vi "AnalysisProcess.vi"(7 "RestartBlocksStates?":bool, 8 "error in (no error)":errorcluster, 9 "Tacho signal In":waveform(dbl), 10 "AccelerationDataIn":waveform(dbl)[](array[waveform]), 11 "QueuesIn":T1) -> (0 "error out":errorcluster, 2 "Tacho signal Out out":waveform(dbl), 3 "AccelerationDataOut out":waveform(dbl)[](array[waveform]))   [LabVIEW 2019]
uses:
  utilities/AQueues.ctl
  AmasterVIs/ACommand.ctl
  AnalyzedVibrationsData.ctl
  AccelerationDataFrames.ctl
  calculateFaultIndicatorsVIs/FaultDetections.ctl
  calculateFaultIndicatorsVIs/ParameterFaultDetection.ctl
  calculateFaultIndicatorsVIs/FaultParameter.ctl
  calculateFaultIndicatorsVIs/FrequencyFaultDetection.ctl
  calculateFaultIndicatorsVIs/OrdersFaultDetection.ctl
  TDMSmanagerVIs/TDMSAnalyzerData.ctl
  TDMSmanagerVIs/TDMSAnalyzerDataType.ctl
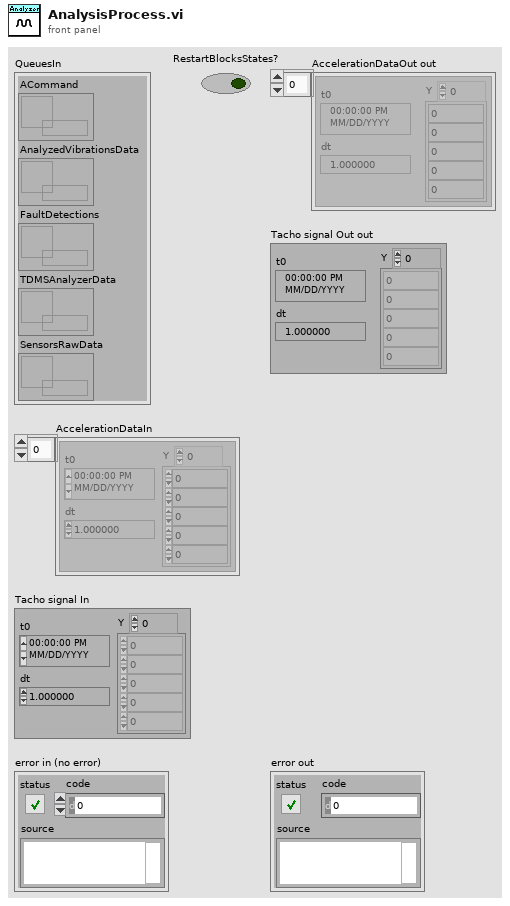
[diagram p1: front panel]
types:
  T1 = typedef "AQueues.ctl" = cluster{"ACommand":refnum<queue>, "AnalyzedVibrationsData":refnum<queue>, "FaultDetections":refnum<queue>, "TDMSAnalyzerData":refnum<queue>, "SensorsRawData":refnum<queue>}
  T2 = typedef "AnalyzerSettings.ctl" = cluster{"Create NS Timeout Code":i32, "Destroy NS Timeout Code":i32, "All threads":T3[], "Connected to app?":bool, "AnalysisSettings":T4}
  T3 = typedef "AThreads.ctl" = enum16{"UI", "analyzeAccelerationData", "aquireAccelerationData", "communicateWebServices", "TDMSmanager", "aquireTachoSignal"}
  T4 = typedef "AnalysisSettings.ctl" = cluster{"Fault Thresholds":T5, "Analysis series name":string, "Save data analysis?":bool, "F-Band Size":i32, "OrderAnalysis?":bool, "Accelerometer":T7, "fs [Hz]":dbl, "Pulse per revolution":u16, "FFT-Parameters":cluster{"averaging mode":enum16{"No averaging", "Vector averaging", "RMS averaging", "Peak hold"}, "weighting mode":enum16{"Linear", "Exponential"}, "number of averages":u32}, "O-WindowPowerSpectrum":u32, "O-SpectrumAveraging":enum16{"No averaging", "Vector averaging", "RMS averaging", "Peak hold"}, "O-MaxOrder":dbl, "O-Resolution":dbl, "O-BandSize":dbl, "FrameLength [s]":dbl, "Aq.FrameLength [ms]":i64, "FilterOrder":i32, "Sensitivity [V/g]":dbl[]}
  T5 = typedef "Thresholds.ctl" = cluster{"Parameters labels":T6[], "Parameters thresholds":dbl[], "Freqs and thresholds":dbl[][], "Orders and thresholds":dbl[][]}
  T6 = typedef "FaultParameter.ctl" = enum16{"Kurtosis", "RMS", "Crest factor"}
  T7 = typedef "Accelerometer.ctl" = enum16{"None", "MPU6050", "MMA7351"}
  T8 = typedef "AccelerationDataFrames.ctl" = cluster{"AccelerationData":waveform(dbl)[], "Amplitudes":cluster{"f0":dbl, "df":dbl, "real part":dbl[]}[], "Phases":cluster{"f0":dbl, "df":dbl, "imaginary part":dbl[]}[]}
  T9 = cluster{"order 0":dbl, "delta order":dbl, "magnitude":dbl[]}[]
  T10 = typedef "svc_Spectrum Info.ctl" = cluster{"channel name":string, "description":string, "x-axis units":T11, "spectral info":cluster{"spectrum type":T12, "linear/dB":enum16{"linear", "dB"}, "window":u16, "window size":i32, "FFT size":i32}, "engineering units":T13, "custom label":string, "dB reference [EU]":dbl, "peak units":enum16{"rms", "peak", "peak-peak"}, "weighting filter":T14, "spectral density?":bool, "unit label":string, "spectrum skewed?":bool, "complimentary spectrum units":T15}
  T11 = typedef "svc_X-Axis Units.ctl" = u16
  T12 = typedef "svc_Spectrum Type.ctl" = enum16{"FFT Spectrum [complex]", "Amplitude [Magnitude]", "Power [Magnitude^2]", "Cross Spectrum [complex]", "Frequency Response [Complex]"}
  T13 = typedef "svc_Engineering Units Text Ring.ctl" = u16
  T14 = typedef "svc_Weighting Filter Text Ring.ctl" = u16
  T15 = typedef "svc_Complimentary Spectrum Units.ctl" = enum16{"none", "radians", "degrees", "cycles", "imaginary"}
  T16 = typedef "OrderAndIndicators.ctl" = cluster{"Order":dbl, "Indicators":dbl[]}
  T17 = typedef "FaultIndicators.ctl" = cluster{"Parameters indicators":dbl[][], "Frequencies indicators":dbl[][]}
  T18 = typedef "FaultDetections.ctl" = cluster{"Parameters fault detection":T19[], "Frequencies fault detection":T20[], "Orders fault detection":T21[]}
  T19 = typedef "ParameterFaultDetection.ctl" = cluster{"Axes Values":dbl[], "Axes Fault Detection":bool[], "Parameter Label":T6}
  T20 = typedef "FrequencyFaultDetection.ctl" = cluster{"Axes Values":dbl[], "Axes Fault Detection":bool[], "Frequency":dbl}
  T21 = typedef "OrdersFaultDetection.ctl" = cluster{"Order":dbl, "Axes Fault Detection":bool[], "Axes Values":dbl[]}
  T22 = typedef "AnalyzedVibrationsData.ctl" = cluster{"AccelerationDataFrames":T8, "Fault detections":T18, "Order Power Spectra":cluster{"order 0":dbl, "delta order":dbl, "magnitude":dbl[]}[], "Tacho signal":waveform(dbl), "Rotational speed [RPM]":dbl}
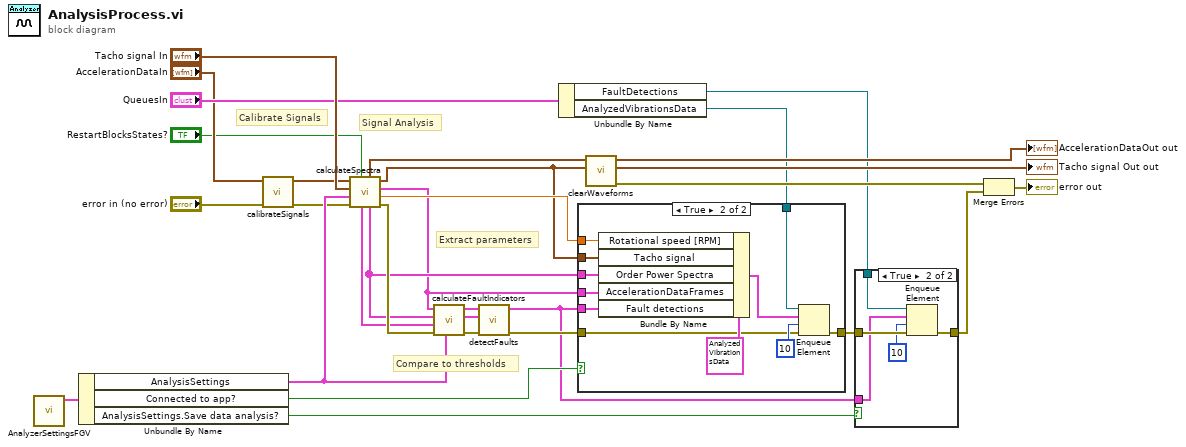
[diagram p0: block diagram]
diagram:
  # "Calibrate Signals"
  # "Compare to thresholds"
  # "Extract parameters"
  # "Signal Analysis"
  n1 = call "AnalyzerSettingsFGV.vi"() -> ("AnalyzerSettingsOut"=w22:T2)  [unwired: 11 in]
  n2 = Unbundle By Name(w22) -> ("AnalysisSettings"=w10:T4, "Connected to app?"=w23:bool, "AnalysisSettings.Save data analysis?"=w24:bool)
  n3 = call "calibrateSignals.vi"("ErrorIn"="error in (no error)", "AccelerationDataIn"="AccelerationDataIn") -> ("ErrorOut"=w5:errorcluster, "AccelerationDataOut"=w2:waveform(dbl)[])  [unwired: 8 in]
  n4 = call "calculateSpectra.vi"("RestartBlocksStates?"="RestartBlocksStates?", "ErrorIn"=w5, "AnalysisSettings"=w10, "Tacho signal In"="Tacho signal In", "AccelerationDataIn"=w2) -> ("ErrorOut"=w31:errorcluster, "Rotational speed [RPM]"=w9:dbl, "AccelerationDataFrames"=w6:T8, "Tacho signal out"=w8:waveform(dbl), "order power spectra"=w7:T9, "AccelerationDataOut"=w26:waveform(dbl)[], "spectrum info"=w30:T10[])
  n5 = call "calculateFaultIndicators.vi"("AnalysisSettings"=w10, "ErrorIn"=w31, "spectrum info"=w30, "order power spectra"=w7, "AccelerationDataFrames"=w6) -> ("ErrorOut"=w29:errorcluster, "Orders and indicators"=w28:T16[], "Fault Indicators"=w27:T17)  [unwired: 4 in]
  n6 = call "detectFaults.vi"("ErrorIn"=w29, "Orders and indicators"=w28, "Fault Indicators"=w27) -> ("ErrorOut"=w20:errorcluster, "Fault detections"=w16:T18)  [unwired: 7 in]
  n7 = Unbundle By Name("QueuesIn") -> ("FaultDetections"=w15:refnum<queue>, "AnalyzedVibrationsData"=w12:refnum<queue>)
  n8 = case shown="True" w23 {
    tunnel: w12 -> [_ w42]
    tunnel: [w32 w41] -> w14
    tunnel: w16 -> [_ w38]
    tunnel: w20 -> [w32 w37]
    tunnel: w9 -> [_ w36]
    tunnel: w8 -> [_ w35]
    tunnel: w7 -> [_ w34]
    tunnel: w6 -> [_ w33]
    frame False {
    }
    frame True {
      n9 = Bundle By Name(cluster=T22 {"AccelerationDataFrames"={"AccelerationData"=[], "Amplitudes"=[], "Phases"=[]}, "Fault detections"={"Parameters fault detection"=[], "Frequencies fault detection"=[], "Orders fault detection"=[]}, "Order Power Spectra"=[], "Tacho signal"={"t0"=timestamp(0 s since 1904-01-01), "dt"=1.0, "Y"=[]}, "Rotational speed [RPM]"=0.0} ("AnalyzedVibrationsData"), "Rotational speed [RPM]"=w36, "Tacho signal"=w35, "Order Power Spectra"=w34, "AccelerationDataFrames"=w33, "Fault detections"=w38) -> (w39:T22)
      n10 = Enqueue Element(queue=w42, element=w39, timeout in ms (-1)=10, error in (no error)=w37) -> (error out=w41:errorcluster)  [unwired: 2 out]
    }
  }
  n11 = call "clearWaveforms.vi"("Tacho signal In"=w8, "AccelerationDataIn"=w26) -> ("ErrorOut"=w17:errorcluster, "Tacho signal Out"=→"Tacho signal Out out":waveform(dbl), "AccelerationDataOut"=→"AccelerationDataOut out":waveform(dbl)[])  [unwired: 7 in]
  n12 = case shown="True" w24 {
    tunnel: w14 -> [w44 w49]
    tunnel: w15 -> [_ w48]
    tunnel: w16 -> [_ w45]
    tunnel: [w44 w47] -> w21
    frame False {
    }
    frame True {
      n13 = Enqueue Element(queue=w48, element=w45, timeout in ms (-1)=10, error in (no error)=w49) -> (error out=w47:errorcluster)  [unwired: 2 out]
    }
  }
  n14 = Merge Errors(w17, w21) -> (→"error out":errorcluster)
